vi "Add_row_to_string_indicator.vi"(3 "show HEX message (T)":bool=TRUE, 6 "string to add":string, 7 "Error string indicator reference":refnum<vi>) -> ()   [LabVIEW 2013]
panel:
  out "String out":string
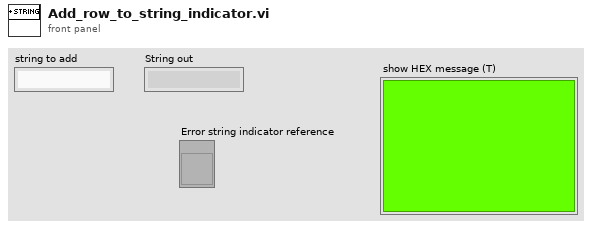
[diagram p1: front panel]
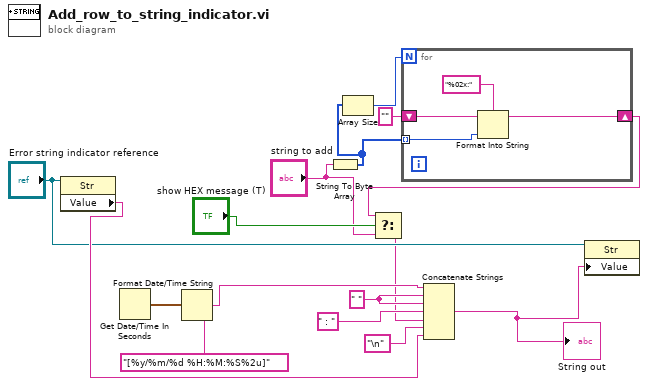
[diagram p0: block diagram]
diagram:
  w8 = " " ("string")
  n1 = property on="Property Node" class="Str"(reference="Error string indicator reference") -> ("Value"=w11:string)  [unwired: 1 in, 2 out]
  n2 = Get Date/Time In Seconds() -> (seconds since 1Jan1904=w14:timestamp)
  n3 = Format Date/Time String(time format string (%c)="[%y/%m/%d %H:%M:%S%2u]", seconds (now)=w14) -> (date/time string=w15:string)  [unwired: 1 in]
  n4 = String To Byte Array(string="string to add") -> (unsigned byte array=w3:u8[])
  n5 = Array Size(array=w3) -> (size(s)=w4:i32)
  n6 = for {
    N: w4 -> [_]
    tunnel: w3 -> [w20] mode=indexing
    shift-right: [w18] -> w1
    shift-left: "" -> [w17]
    n7 = Format Into String(format string="%02x:", initial string=w17, w20) -> (resulting string=w18:string)  [unwired: 1 in, 1 out]
  }
  n8 = Select(t=w1, s="show HEX message (T)", f="string to add") -> (s? t:f=w6:string)
  n9 = Concatenate Strings(w15, w8, w8, " : " ("string"), w6, "\n" ("string"), w11) -> (w10:string)
  "String out" <- w10
  n10 = property on="Property Node" class="Str"(reference="Error string indicator reference", "Value"=w10) -> ()  [unwired: 1 in, 2 out]
